vi "DFD Non-Uniform Filter Bank Reconstruction (Array).vi"(7 "init? (F)":bool, 8 "error in (no error)":errorcluster, 10 "filter bank in":T1 {"mFBank_SynthesisFilters"."mMRate_SumWl" min=1 max=32 step=1; "mFBank_SynthesisFilters"."mMRate_InputIwl" min=1 max=32 step=1; "mFBank_SynthesisFilters"."mMRate_GainWl" min=1 max=32 step=1; "mFBank_SynthesisFilters"."mMRate_OutputWl" min=1 max=32 step=1; "mFBank_SynthesisFilters"."mMRate_InputWl" min=1 max=32 step=1; "mFBank_SynthesisFilters"."mMRate_CoefWl" min=1 max=32 step=1; "mFBank_SynthesisFilters"."mMRate_Mode" items=["Default"=-1, "No Rate Change"=0, "Interpolation"=1, "Decimation"=2, "Interpolated"=3, "Rational"=4]; "mFBank_AnalysisFilters"."mMRate_SumWl" min=1 max=32 step=1; "mFBank_AnalysisFilters"."mMRate_InputIwl" min=1 max=32 step=1; "mFBank_AnalysisFilters"."mMRate_GainWl" min=1 max=32 step=1; "mFBank_AnalysisFilters"."mMRate_OutputWl" min=1 max=32 step=1; "mFBank_AnalysisFilters"."mMRate_InputWl" min=1 max=32 step=1; "mFBank_AnalysisFilters"."mMRate_CoefWl" min=1 max=32 step=1; "mFBank_AnalysisFilters"."mMRate_Mode" items=["Default"=-1, "No Rate Change"=0, "Interpolation"=1, "Decimation"=2, "Interpolated"=3, "Rational"=4]; "mFBank_Type" items=["Uniform", "Non-Uniform"]}, 11 "M bands":cluster{"Array":dbl[]}[](array[cluster])) -> (0 "error out":errorcluster, 3 "y":dbl[](array[numeric]))   [LabVIEW 2023]
doc: "Reconstructs signal from M-channel sequences <B>x</B> using an M-band synthesis bank specified by <B>synthesis bank</B> continuously. The initial internal states are controlled by <B>init? (F)</B>.\n\nYou can call the VIs in <B>Filter Bank Design</B> sub-palette to design a filter bank."
uses:
  <vilib>/addons/Digital Filter Design/FilterBank.llb/Object/DFD Filter Bank Obj.ctl
  <vilib>/addons/Digital Filter Design/_Objects.llb/DFD Multirate Filter Obj.ctl
  <vilib>/addons/Digital Filter Design/_Objects.llb/DFD Multirate Mode.ctl
  <vilib>/addons/Digital Filter Design/_Objects.llb/DFD Coef Norm Type.ctl
  <vilib>/addons/Digital Filter Design/_Objects.llb/DFD Round-off Mode.ctl
  <vilib>/addons/Digital Filter Design/_Objects.llb/DFD FXP MRate Multiply Mode.ctl
  <vilib>/addons/Digital Filter Design/FilterBank.llb/Object/DFD Filter Bank Processing Method.ctl
  <vilib>/addons/Digital Filter Design/FilterBank.llb/Object/DFD Filter Bank Type.ctl
  <vilib>/addons/Digital Filter Design/Multirate.llb/DFD MRate Filtering with State (Array).vi
  <vilib>/addons/Digital Filter Design/Process.llb/DFD Integer Delay (Array).vi
  <vilib>/addons/Digital Filter Design/NI_DigFilterLicensed.lvlib
  <vilib>/addons/Digital Filter Design/NI_DigFilter_FilterBank.lvlib
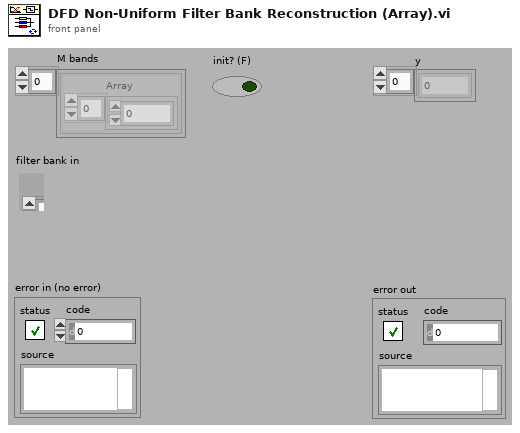
[diagram p1: front panel]
types:
  T1 = typedef "NI_DigFilter_FilterBank.lvlib/DFD Filter Bank Obj.ctl" = cluster{"mFBank_AnalysisFilters":T2[], "mFBank_SynthesisFilters":T2[], "mFBank_#Bands":i32, "mFBank_ProcMethod":T7, "mFBank_Coeffs":dbl[], "mFBank_Gain":dbl, "mFBank_Delay":i32, "mFBank_Type":T8}
  T2 = typedef "NI_DigFilterLicensed.lvlib/DFD Multirate Filter Obj.ctl" = cluster{"mMRate_Structure":enum16{"CIC", "FIR", "IIR", "Lattice"}, "mMRate_Mode":T3, "mMRate_Factor":i32, "mMRate_FIRParams":cluster{"mMRate_FIR_H":dbl[], "mMRate_FIR_IsNyquist?":bool, "mMRate_FIR_IsSymmetric?":bool}, "mMRate_CICParams":cluster{"mMRate_CIC_#Stage":i32, "mMRate_CIC_Lag":i32, "mMRate_CIC_Type":enum16{"Lowpass", "Highpass"}}, "mMRate_Order":i32, "mMRate_Version":string, "mMRate_Comments":string, "mMRate_RationalFactor":cluster{"mMRate_L":i32, "mMRate_M":i32}, "mMRate_Fs":dbl, "mMRate_Quantized?":bool, "mMRate_QFilterGain":dbl, "mMRate_CoefWl":i16, "mMRate_Scaling":cluster{"mMRate_ScaleByPowerOf2?":bool, "mMRate_ScaleType":T4}, "mMRate_InputWl":i16, "mMRate_OutputWl":i16, "mMRate_OutputMode":T5, "mMRate_MultMode":T6, "mMRate_BitPruning":bool, "mMRate_GainWl":i16, "mMRate_OutputFwl":i16, "mMRate_SumIwl":i16, "mMRate_InputIwl ":i16, "mMRate_SumWl":i16, "mMRate_CoefIwl":i16}
  T3 = typedef "NI_DigFilterLicensed.lvlib/DFD Multirate Mode.ctl" = i16
  T4 = typedef "NI_DigFilterLicensed.lvlib/DFD Coef Norm Type.ctl" = enum16{"No Norm", "Time Domain 1-Norm", "Time Domain 2-Norm", "Time Domain Inf-Norm"}
  T5 = typedef "NI_DigFilterLicensed.lvlib/DFD Round-off Mode.ctl" = enum16{"Nearest", "Truncation"}
  T6 = typedef "NI_DigFilterLicensed.lvlib/DFD FXP MRate Multiply Mode.ctl" = enum16{"Truncated", "Full"}
  T7 = typedef "NI_DigFilter_FilterBank.lvlib/DFD Filter Bank Processing Method.ctl" = enum16{"General", "2-Band QMF Lattice", "Cosine-Modulated"}
  T8 = typedef "NI_DigFilter_FilterBank.lvlib/DFD Filter Bank Type.ctl" = u16
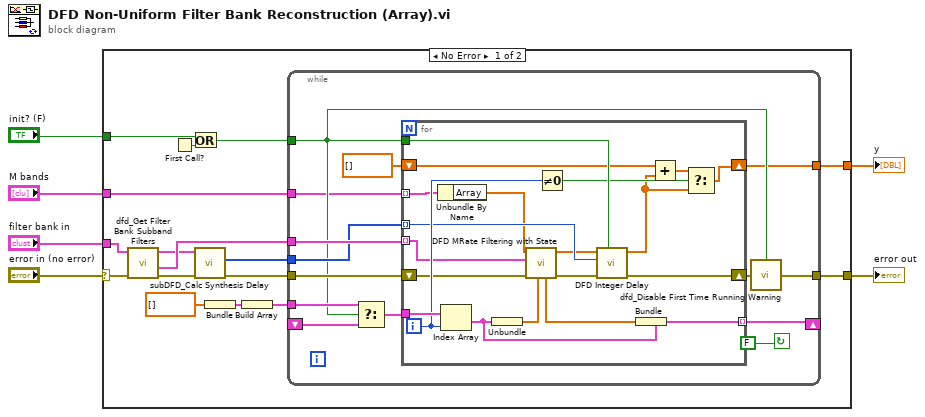
[diagram p0: block diagram]
diagram:
  n1 = case shown="No Error" "error in (no error)" {
    selector: "error in (no error)" -> [w13 w57]
    tunnel: "filter bank in" -> [w14 _]
    tunnel: "M bands" -> [w11 _]
    tunnel: [w19 w57] -> w2
    tunnel: "init? (F)" -> [w17 _]
    tunnel: [w12 _] -> w1
    frame No Error {
      n2 = call <vilib>:"dfd_Get Filter Bank Subband Filters.vi"("error in (no error)"=w13, "filter bank in"=w14) -> ("error out"=w10:errorcluster, "synthesis filters"=w15:T2[], "filter bank out"=w9:T1)  [unwired: 6 in, 1 out]
      n3 = First Call?() -> (First Call?: T/F=w16:bool)
      n4 = Or(x=w17, y=w16) -> (x .or. y?=w18:bool)
      n5 = call "subDFD_Calc Synthesis Delay.vi"("error in (no error)"=w10, "tree in"=w9) -> ("error out"=w7:errorcluster, "syn_delay"=w8:i32[])  [unwired: 7 in, 1 out]
      n6 = Bundle(dbl[] []) -> (w21:cluster{dbl[]})  [unwired: 1 in]
      n7 = Build Array(w21) -> (w20:cluster{dbl[]}[])
      n8 = while {
        tunnel: w15 -> [w29]
        tunnel: w7 -> [w30]
        shift-right: [w31] -> _
        shift-left: _ -> [w35]
        tunnel: w18 -> [w26]
        tunnel: w20 -> [w36]
        tunnel: [w33] -> w19
        tunnel: w8 -> [w27]
        tunnel: [w25] -> w12
        tunnel: w11 -> [w23]
        stop <- FALSE continue-if-true
        n9 = Select(t=w36, s=w26, f=w35) -> (s? t:f=w32:cluster{dbl[]}[])
        n10 = for {
          tunnel: w29 -> [w45] mode=indexing
          shift-right: [w40] -> w28
          shift-left: w30 -> [w42]
          tunnel: w32 -> [w50]
          tunnel: [w53] -> w31 mode=indexing
          shift-right: [w47] -> w25
          shift-left: dbl[] [] ("signal out") -> [w51]
          tunnel: w27 -> [w44] mode=indexing
          tunnel: w26 -> [w52]
          tunnel: w23 -> [w43] mode=indexing
          i -> [w49]
          n11 = Unbundle By Name(w43) -> ("Array"=w38:dbl[])
          n12 = Index Array(array=w50, index=w49) -> (element=w54:cluster{dbl[]})
          n13 = Unbundle(w54) -> (w55:dbl[])
          n14 = call-poly <vilib>:"DFD MRate Filtering with State.vi"("state in"=w55, "error in (no error)"=w42, "multirate filter"=w45, "signal in"=w38) -> ("error out"=w41:errorcluster, "signal out"=w39:dbl[], "state out"=w56:dbl[])  [unwired: 5 in]
          n15 = Not Equal To 0?(x=w49) -> (x != 0?=w48:bool)
          n16 = call-poly <vilib>:"DFD Integer Delay.vi"("init? (F)"=w52, "error in (no error)"=w41, "delay"=w44, "signal in"=w39) -> ("error out"=w40:errorcluster, "signal out"=w37:dbl[])  [unwired: 6 in]
          n17 = Bundle(cluster=w54, w56) -> (w53:cluster{dbl[]})
          n18 = Add(x=w51, y=w37) -> (x+y=w46:dbl[])
          n19 = Select(t=w46, s=w48, f=w37) -> (s? t:f=w47:dbl[])
        }
        n20 = call <vilib>:"dfd_Disable First Time Running Warning.vi"("error in"=w28, "disable?"=w26) -> ("error out"=w33:errorcluster)
      }
    }
    frame Error {
    }
  }
  "error out" <- w2
  "y" <- w1
